vi "Jump to Next.vi"(8 "error in (no error)":errorcluster, 11 "BaseProducer in":refnum<class "BaseProducer.lvclass">) -> (0 "error out":errorcluster, 3 "BaseProducer out":refnum<class "BaseProducer.lvclass">)   [LabVIEW 2013, in "BaseProducer.lvclass"]
doc: "This method jumps straight to its input state, monitoring sensors for blowout and exiting when the state is reached."
uses:
  BaseProducer.lvclass
  <vilib>/DAQmx/read.llb/DAQmx Read (Analog 1D DBL NChan 1Samp).vi
  <vilib>/DAQmx/write.llb/DAQmx Write (Analog 1D DBL NChan 1Samp).vi
panel:
  in  "Skip":bool
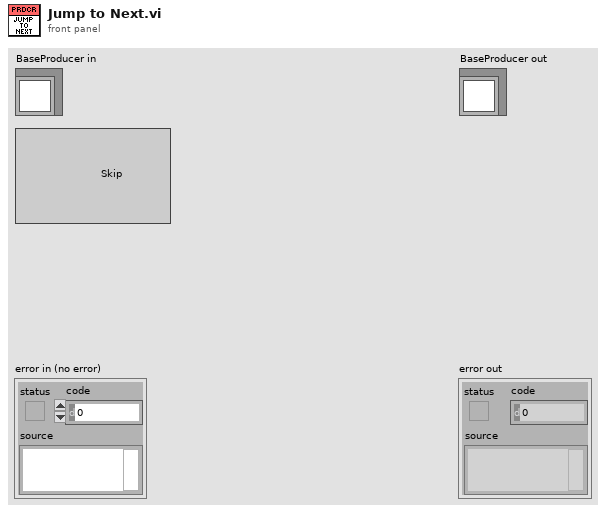
[diagram p1: front panel]
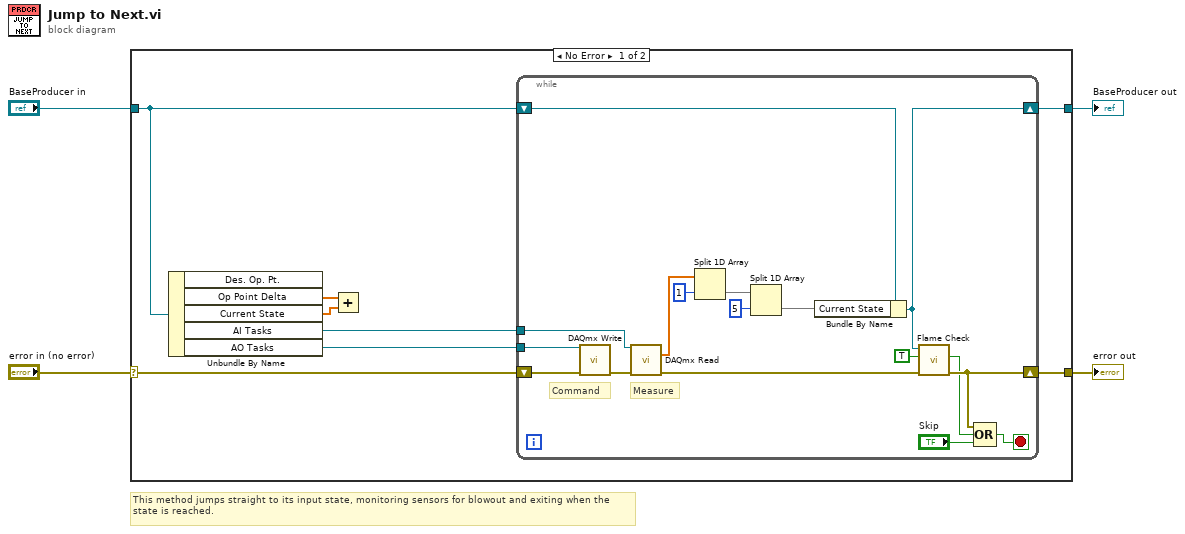
[diagram p0: block diagram]
diagram:
  # "This method jumps straight to its input state, monitoring sensors for blowout and exiting when the state is reached."
  n1 = case shown="No Error" "error in (no error)" {
    selector: "error in (no error)" -> [w11 w31]
    tunnel: [w10 w31] -> w3
    tunnel: [w12 w30] -> w1
    tunnel: "BaseProducer in" -> [w5 w30]
    frame No Error {
      n2 = Unbundle By Name(w5) -> ("Op Point Delta"=w6:dbl[], "Current State"=w7:dbl[], "AI Tasks"=w8:refnum<k21>, "AO Tasks"=w9:refnum<k21>)  [unwired: 1 out]
      n3 = Add(x=w6, y=w7) -> ()  [unwired: 1 out]
      n4 = while {
        shift-right: [w14] -> w12
        shift-left: w5 -> [w15]
        shift-right: [w24] -> w10
        shift-left: w11 -> [w28]
        tunnel: w9 -> [w21]
        tunnel: w8 -> [w20]
        stop <- w22 stop-if-true
        # "Measure"
        # "Command"
        n5 = call-poly <vilib>:"DAQmx Write.vi"("task/channels in"=w21, "error in"=w28) -> ("error out"=w29:errorcluster)  [unwired: 11 in, 2 out]
        n6 = call-poly <vilib>:"DAQmx Read.vi"("task/channels in"=w20, "error in"=w29) -> ("data"=w16:dbl[], "error out"=w27:errorcluster)  [unwired: 11 in, 1 out]
        n7 = Split 1D Array(array=w16, index=1) -> (second subarray=w18:dbl[])  [unwired: 1 out]
        n8 = Split 1D Array(array=w18, index=5) -> (second subarray=w13:dbl[])  [unwired: 1 out]
        n9 = Bundle By Name(cluster=w15, "Current State"=w13) -> (w14:refnum<class "BaseProducer.lvclass">)
        n10 = call "Flame Check.vi"("error in (no error)"=w27, "Resample? (F)"=TRUE, "BaseProducer in"=w14) -> ("error out"=w24:errorcluster, "Flame?"=w23:bool)  [unwired: 6 in, 1 out]
        n11 = Compound Arithmetic op=OR(w24, w23, "Skip") -> (w22:bool)
      }
    }
    frame Error {
    }
  }
  "error out" <- w3
  "BaseProducer out" <- w1
